vi "dort_islem_kullanıldı.vi"() -> ()   [LabVIEW 2019]
panel:
  in  "Sayi2":string
  in  "Sayi1":string
  out "Sonuç":dbl
  in  "Ýþlem türü":string
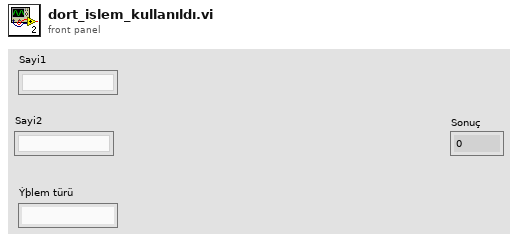
[diagram p1: front panel]
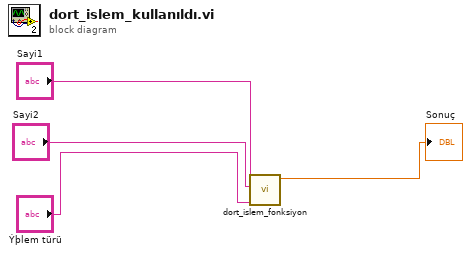
[diagram p0: block diagram]
diagram:
  n1 = call "dort_islem_fonksiyon.vi"("Ýþlem"="Ýþlem türü", "Sayi2"="Sayi2", "Sayi1"="Sayi1") -> ("Sonuç"=→"Sonuç":dbl)  [unwired: 8 in]
